vi "UI Help.vi"(8 "error in (no error)":errorcluster) -> (0 "error out":errorcluster)   [LabVIEW 2016]
doc: "Help for User Interface"
panel:
  # "Image Analyzer"
  # "[Click anywhere in this to close the Help]"
  # "Objective:\nThis application allows users to perform some basic operations on the acquired image and help users to understand the\nimage processing concepts."
  # "Instructions:\n1. Make sure at least one camera  or Framegrabber or any IMAQdx compatible device is connected to the system.\n\n2. Choose the valid camera using the Choose Camera option.\n\n3. Now click on the Start Acquisition button to view the Live Feed from the chosen device.\n\n4. Now click on any one of the operations listed under Operations Available.\n     Note: You can click on various operations mulple times. Each time user clicks on the available operation, A new\n              window will be opened appropriately. User can work on multiple operations in parallel.\n\n5. Once the operation is understood, user can close the appropriate window. \n\n6.  To stop the acquisition, click on the Stop Acquisition button. This will stop the Live Feed from device."
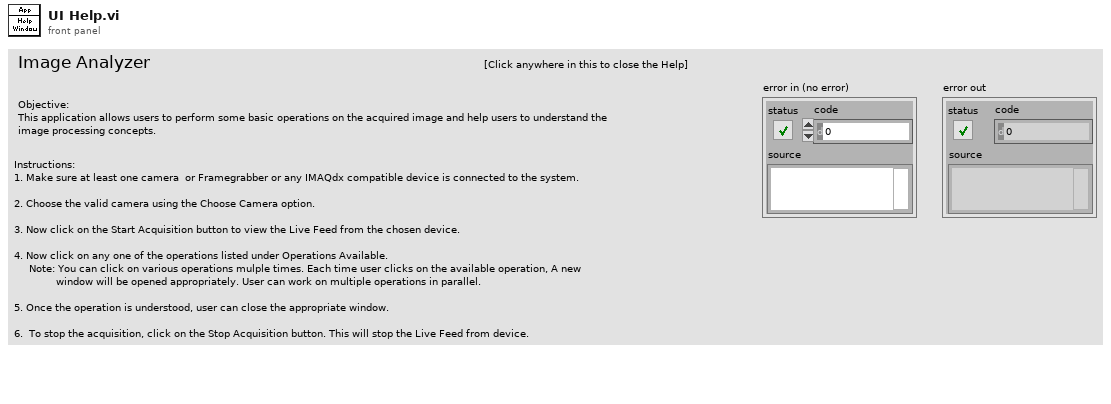
[diagram p1: front panel]
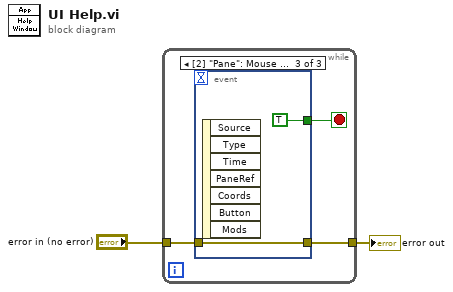
[diagram p0: block diagram]
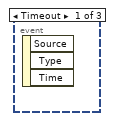
[diagram p2: hidden frame]
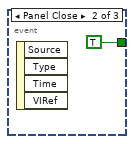
[diagram p3: hidden frame]
diagram:
  n1 = while {
    tunnel: "error in (no error)" -> [w4]
    tunnel: [w3] -> w1
    stop <- w5 stop-if-true
    n2 = event shown="[2] \"Pane\": Mouse Down" {
      selector: _ -> [_ _ _]
      dyn-events: _ -> [_ _ _]
      timeout: _ -> [_ _ _]
      tunnel: [_ TRUE TRUE] -> w5
      tunnel: w4 -> [_ _ w7]
      tunnel: [_ _ w7] -> w3
      event Timeout {
        n3 = event-data() -> ()  [unwired: 1 in, 3 out]
      }
      event Panel Close {
        n4 = event-data() -> ()  [unwired: 1 in, 4 out]
      }
      event Mouse Down {
        n5 = event-data() -> ()  [unwired: 1 in, 7 out]
      }
    }
  }
  "error out" <- w1
